vi "Update Channel Selectors.vi"(8 "error in (no error)":errorcluster, 11 "XY WFRM Plot in":refnum<class "XY WFRM Plot.lvclass">) -> (0 "error out":errorcluster, 3 "XY WFRM Plot out":refnum<class "XY WFRM Plot.lvclass">)   [LabVIEW 2019, in "XY WFRM Plot.lvclass"]
uses:
  XY WFRM Plot.lvclass
  C:/GitHub/LabActor/Plots/Plot/Plot.lvclass
  Plot/Plot.lvclass/Plot.ctl
  XY WFRM Plot.lvclass/XY WFRM Plot.ctl
  Plot/Read Files.vi
  Read X column ref.vi
  Read Y columns ref.vi
  Plot/Plot.lvclass
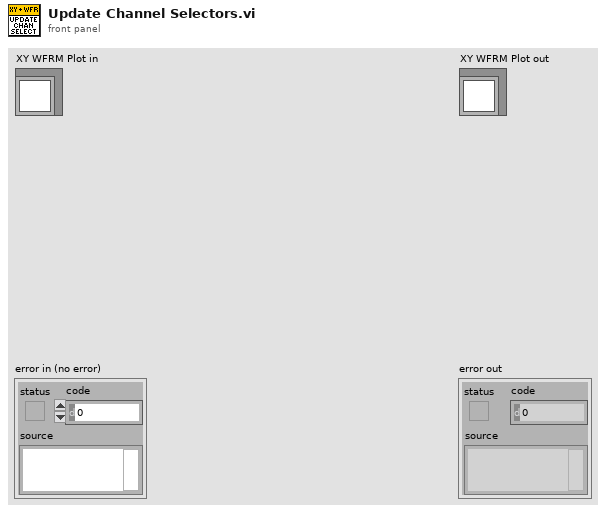
[diagram p1: front panel]
types:
  T1 = typedef "File_Group_Chan_Abbr.ctl" = cluster{"File Path Control":path, "Group":string, "Channel":string, "Abbreviated":string}
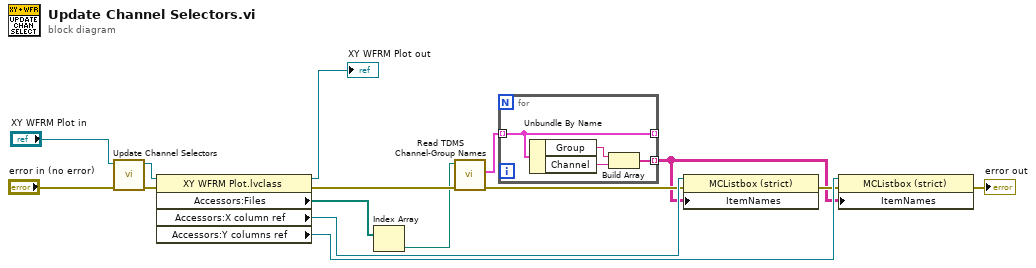
[diagram p0: block diagram]
diagram:
  n1 = call-parent "Update Channel Selectors.vi"("error in (no error)"="error in (no error)", "Plot in"="XY WFRM Plot in") -> ("error out"=w13:errorcluster, "Plot out"=w12:refnum<class "XY WFRM Plot.lvclass">)  [unwired: 8 in]
  n2 = property class="XY WFRM Plot.lvclass"(reference=w12, error in=w13) -> (reference out=→"XY WFRM Plot out":refnum<class "XY WFRM Plot.lvclass">, error out=w11:errorcluster, "Accessors:Files"=w10:path[], "Accessors:X column ref"=w7:refnum<vi>, "Accessors:Y columns ref"=w6:refnum<vi>)
  n3 = Index Array(array=w10) -> (element=w9:path)  [unwired: 1 in]
  n4 = call "Read TDMS Channel-Group Names.vi"("error in"=w11, "File Path Control"=w9) -> ("error out"=w5:errorcluster, "File-group-channel"=w8:T1[])  [unwired: 8 in]
  n5 = for {
    tunnel: [w19] -> _ mode=indexing
    tunnel: w8 -> [w19] mode=indexing
    tunnel: [w16] -> w3 mode=indexing
    n6 = Unbundle By Name(w19) -> ("Group"=w18:string, "Channel"=w17:string)
    n7 = Build Array(w18, w17) -> (w16:string[])
  }
  n8 = property class="MCListbox (strict)"(reference=w7, error in=w5, "ItemNames"=w3) -> (error out=w4:errorcluster)  [unwired: 1 out]
  n9 = property class="MCListbox (strict)"(reference=w6, error in=w4, "ItemNames"=w3) -> (error out=→"error out":errorcluster)  [unwired: 1 out]
